vi "DB init.vi"(8 "error in (no error)":errorcluster, 11 "DB path":path) -> (0 "error out":errorcluster, 3 "DB Data":T1)   [LabVIEW 2020]
uses:
  <vilib>/drjdpowell/SQLite Library/SQL Connection/Open (path).vi
  <vilib>/drjdpowell/SQLite Library/SQL Connection/Open (string).vi
  <vilib>/AdvancedString/Path To Command Line String.vi
  <vilib>/drjdpowell/SQLite Library/SQL Connection/Execute SQL.vi
  <vilib>/drjdpowell/SQLite Library/SQL Connection/Connection.lvclass
  <vilib>/drjdpowell/SQLite Library/SQLite.lvlib
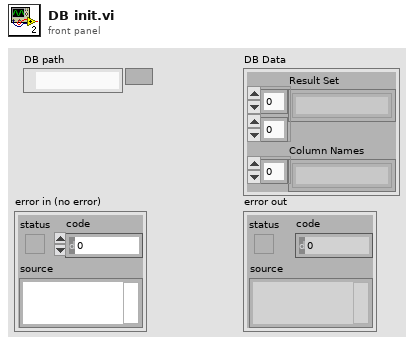
[diagram p1: front panel]
types:
  T1 = cluster{"Result Set":string[][], "Column Names":string[]}
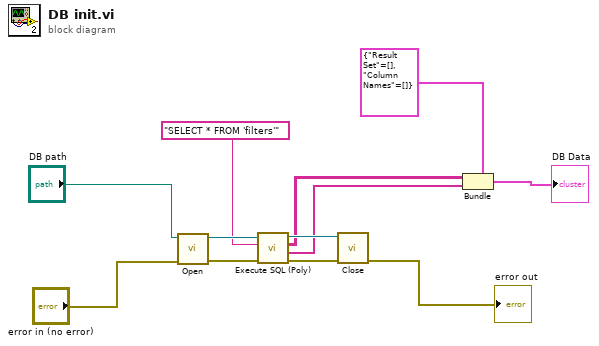
[diagram p0: block diagram]
diagram:
  n1 = call-poly <vilib>:"Open.vi"("error in (no error)"="error in (no error)", "db file"="DB path") -> ("error out"=w10:errorcluster, "SQLite Connection"=w12:refnum<class "Connection.lvclass">)  [unwired: 8 in]
  n2 = call-poly <vilib>:"Execute SQL (Poly).vi"("error in (no error)"=w10, "SQL"="SELECT * FROM 'filters'", "SQLite Connection in"=w12) -> ("error out"=w9:errorcluster, "Column Names"=w4:string[], "Result Set"=w5:string[][], "SQLite Connection"=w7:refnum<class "Connection.lvclass">)  [unwired: 5 in]
  n3 = call-dynamic "Close.vi"("error in (no error)"=w9, "SQLite Connection in"=w7) -> ("error out"=→"error out":errorcluster)  [unwired: 9 in]
  n4 = Bundle(cluster=T1 {"Result Set"=[], "Column Names"=[]}, "Result Set"=w5, "Column Names"=w4) -> (→"DB Data":T1)
